vi "Dpc Put Tdi Bits.vi"(0 "hif":u32, 1 "cbit":i32, 2 "rgbSnd":string, 3 "bitTms":i32, 4 "fReturnTdo":i32, 5 "rgbRcv":string, 6 "perc":i32, 7 "error in (no error)":errorcluster, 8 "ptrid":u16) -> (18 "ptrid out":u16, 20 "hif out":u32, 21 "function return":i32, 22 "rgbSnd out":string, 25 "rgbRcv out":string, 26 "perc out":i32, 27 "error out":errorcluster)   [LabVIEW 2011, in "LVH-Adept.lvlib" / "DPCUTIL.lvlib"]
doc: "DPCAPI BOOL DpcPutTdiBits(HANDLE hif, INT32 cbit, BYTE * rgbSnd, BOOL bitTms, BOOL fReturnTdo, BYTE * rgbRcv, ERC * perc, TRID * ptrid);"
uses:
  DPCUTIL.lvlib
  dpcutil.dll
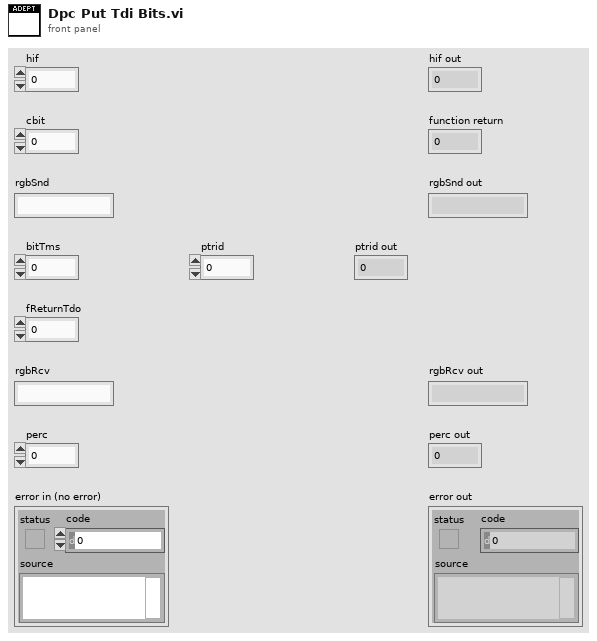
[diagram p1: front panel]
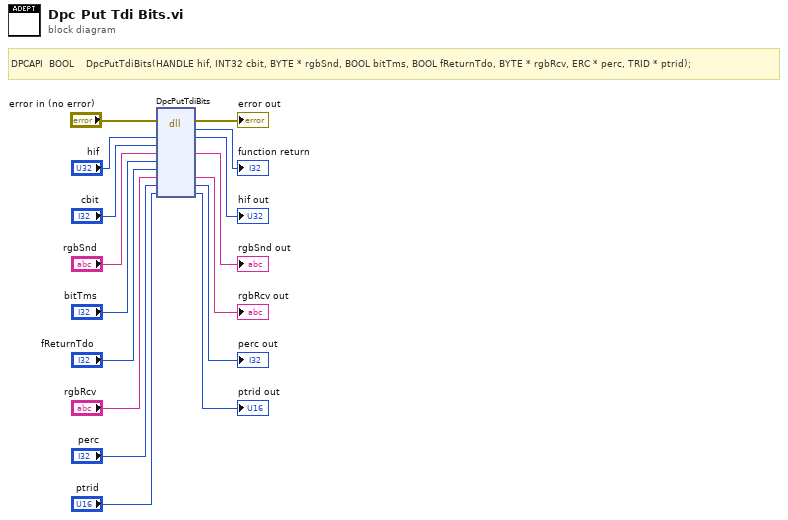
[diagram p0: block diagram]
diagram:
  # "DPCAPI  BOOL    DpcPutTdiBits(HANDLE hif, INT32 cbit, BYTE * rgbSnd, BOOL bitTms, BOOL fReturnTdo, BYTE * rgbRcv, ERC * perc, TRID * ptrid);"
  n1 = dll-call lib="dpcutil.*" fn="DpcPutTdiBits"(error in="error in (no error)", "hif"="hif", "cbit"="cbit", "rgbSnd"="rgbSnd", "bitTms"="bitTms", "fReturnTdo"="fReturnTdo", "rgbRcv"="rgbRcv", "perc"="perc", "ptrid"="ptrid") -> (error out=→"error out":errorcluster, →"function return":i32, "hif"=→"hif out":u32, "rgbSnd"=→"rgbSnd out":string, "rgbRcv"=→"rgbRcv out":string, "perc"=→"perc out":i32, "ptrid"=→"ptrid out":u16)  [unwired: 5 in, 1 out]
